vi "FTW-ERR-SourceLevelIncrement.vi"(1 "SourceLevelIn":i32) -> (0 "SourceLevelOut":i32)   [LabVIEW 2018]
doc: "Increments source level\n\nThis VI is for private use only"
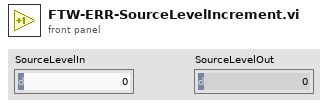
[diagram p1: front panel]
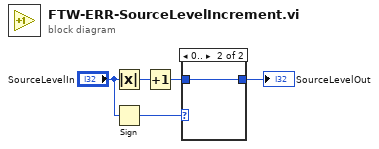
[diagram p0: block diagram]
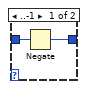
[diagram p2: hidden frame]
diagram:
  n1 = Absolute Value(x="SourceLevelIn") -> (abs(x)=w5:i32)
  n2 = Sign(1:"SourceLevelIn") -> (0:w3:i32)
  n3 = Increment(x=w5) -> (x+1=w2:i32)
  n4 = case shown="0.." w3 {
    tunnel: w2 -> [w7 w8]
    tunnel: [w6 w8] -> w1
    frame ..-1 {
      n5 = Negate(x=w7) -> (-x=w6:i32)
    }
    frame 0.. {
    }
  }
  "SourceLevelOut" <- w1
